vi "Stop Core.vi"(10 "final error code":i32, 11 "Nested in":refnum<class "Database Provider.lvclass">) -> (3 "Nested out":refnum<class "Database Provider.lvclass">)   [LabVIEW 2024, in "Database Provider.lvlib" / "Database Provider.lvclass"]
doc: "(<B>Filename</B>: Actor Framework.lvlib:Actor.lvclass:Stop Core.vi)\n\nDefines what the actor does before it stops. Use the <B>final error code</B> input to determine whether the actor shut down in response to an error.\n\nBy default, this method does nothing. A descendant class may override it to define behavior, such as shutting down any processes the actor initiated in its override of the Actor Core method."
uses:
  Database Provider.lvclass
  Database Provider.lvclass/Database Provider.ctl
  <vilib>/MGI/Panel Manager/Panel Actor/Panel Actor/Panel Actor.lvclass
  <vilib>/drjdpowell/SQLite Library/SQL Connection/Connection.lvclass
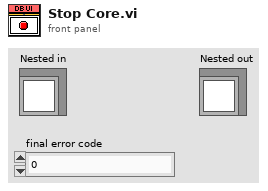
[diagram p1: front panel]
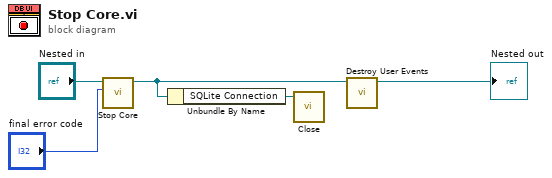
[diagram p0: block diagram]
diagram:
  n1 = call-parent "Stop Core.vi"("final error code"="final error code", "Actor in"="Nested in") -> ("Actor out"=w2:refnum<class "Database Provider.lvclass">)  [unwired: 9 in]
  n2 = Unbundle By Name(w2) -> ("SQLite Connection"=w1:refnum<class "Connection.lvclass">)
  n3 = call-dynamic "Close.vi"("SQLite Connection in"=w1) -> ()  [unwired: 10 in, 1 out]
  n4 = call "Destroy User Events.vi"("UI Template in"=w2) -> ("UI Template out"=→"Nested out":refnum<class "Database Provider.lvclass">)  [unwired: 10 in]
